vi "ExtractArchivedSpectra.vi"() -> ()   [LabVIEW 2013, in "examples.lvlib"]
uses:
  examples.lvlib
  vis/lv-2013/tango_vi.llb/avToDoubleSpectrumAv.vi
  vis/lv-2013/tango_vi.llb/tango.lvlib
panel:
  out "success":bool
  out "Intensity Chart":dbl[][](graph)
  out "timestamps":dbl[](array[numeric])
  out "archived sprectra":dbl[][](array[numeric])
  in  "sampling":string="MINUTE"
  in  "to_date":string="2010-02-02 00:00:00"
  in  "from_date":string="2010-02-01 00:00:00"
  in  "archived_attr_name":string="ANS-C03/DG/DCCT/current"
  in  "db_extractor_dev_name":string="archiving/hdbextractor/1"
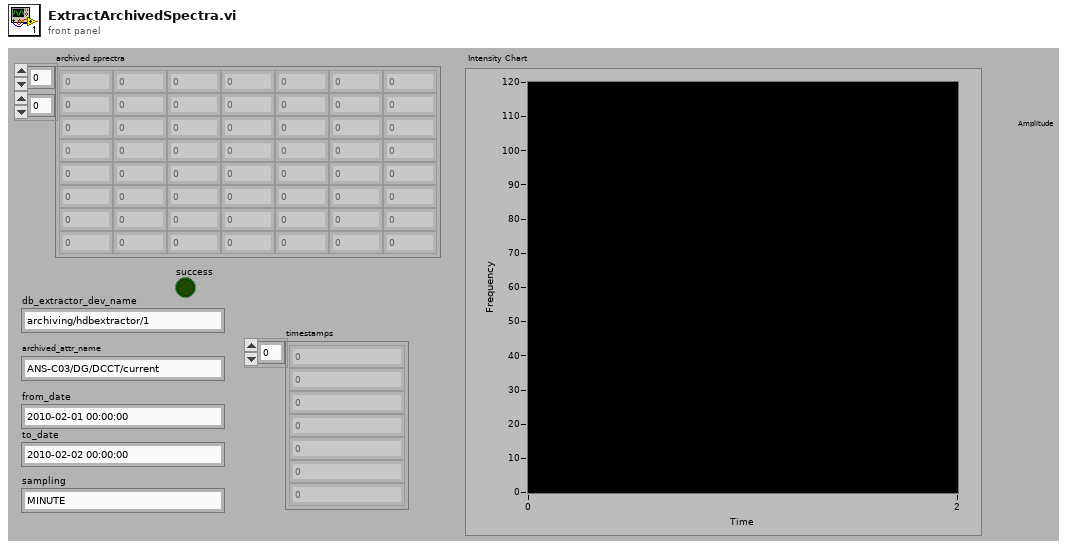
[diagram p1: front panel]
types:
  T1 = cluster{"device name":string, "attribute name":string, "quality value":i16, "quality string":string, "timestamp":dbl, "dim. x":i32, "dim. y":i32, "value":u8[], "error code":i32, "error stack":string[], "data type":u16}[]
  T2 = cluster{"device name":string, "attribute name":string, "quality value":i16, "quality string":string, "timestamp":dbl, "dim. x":i32, "dim. y":i32, "value":dbl[], "error code":i32, "error stack":string[], "data type":u16}
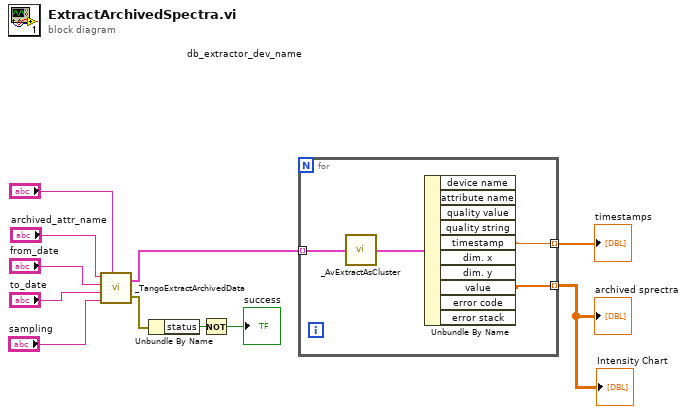
[diagram p0: block diagram]
diagram:
  n1 = call "_TangoExtractArchivedData.vi"("db_extractor_dev_name"="db_extractor_dev_name", "sampling"="sampling", "to_date"="to_date", "from_date"="from_date", "archived_attr_name"="archived_attr_name") -> ("error out"=w1:errorcluster, "attr values"=w6:T1)  [unwired: 1 in]
  n2 = Unbundle By Name(w1) -> ("status"=w3:bool)
  n3 = Not(x=w3) -> (.not. x?=→"success":bool)
  n4 = for {
    tunnel: w6 -> [w15] mode=indexing
    tunnel: [w13] -> w5 mode=indexing
    tunnel: [w12] -> w4 mode=indexing
    n5 = call-poly "_AvExtractAsCluster.vi"("attribute value"=w15) -> ("av"=w14:T2)
    n6 = Unbundle By Name(w14) -> ("timestamp"=w13:dbl, "value"=w12:dbl[])  [unwired: 8 out]
  }
  "archived sprectra" <- w4
  "timestamps" <- w5
  "Intensity Chart" <- w4
